vi "test4.3-AsyncMessageWithoutReply_Queue.vi"(8 "error in (no error)":errorcluster, 11 "TestCase in":refnum<class "testcase-CSMGlobalLog.lvclass">) -> (0 "error out":errorcluster, 3 "TestCase out":refnum<class "testcase-CSMGlobalLog.lvclass">)   [LabVIEW 2017, in "testcase-CSMGlobalLog.lvclass"]
uses:
  testcase-CSMGlobalLog.lvclass
  testcase-CSMGlobalLog.lvclass/testcase-CSMGlobalLog.ctl
  c9cb4a92-c6b2-48ff-9945-b938079fd949.vi
  <vilib>/addons/_JKI Toolkits/VI Tester/TestCase.llb/TestCase.lvclass
  src/user.lib/_NEVSTOP/Communicable State Machine(CSM)/Communicable State Machine.lvlib
  src/user.lib/_NEVSTOP/Communicable State Machine(CSM)/Utility/Periodic String Filter Setting.ctl
  C:/Program Files (x86)/National Instruments/LabVIEW 2017/vi.lib/addons/_JKI Toolkits/VI Tester/TestCase.llb/TestCase.lvclass
panel:
  out "String cache total":string
  out "LoopCount":i32
  out "String Cache each loop":string
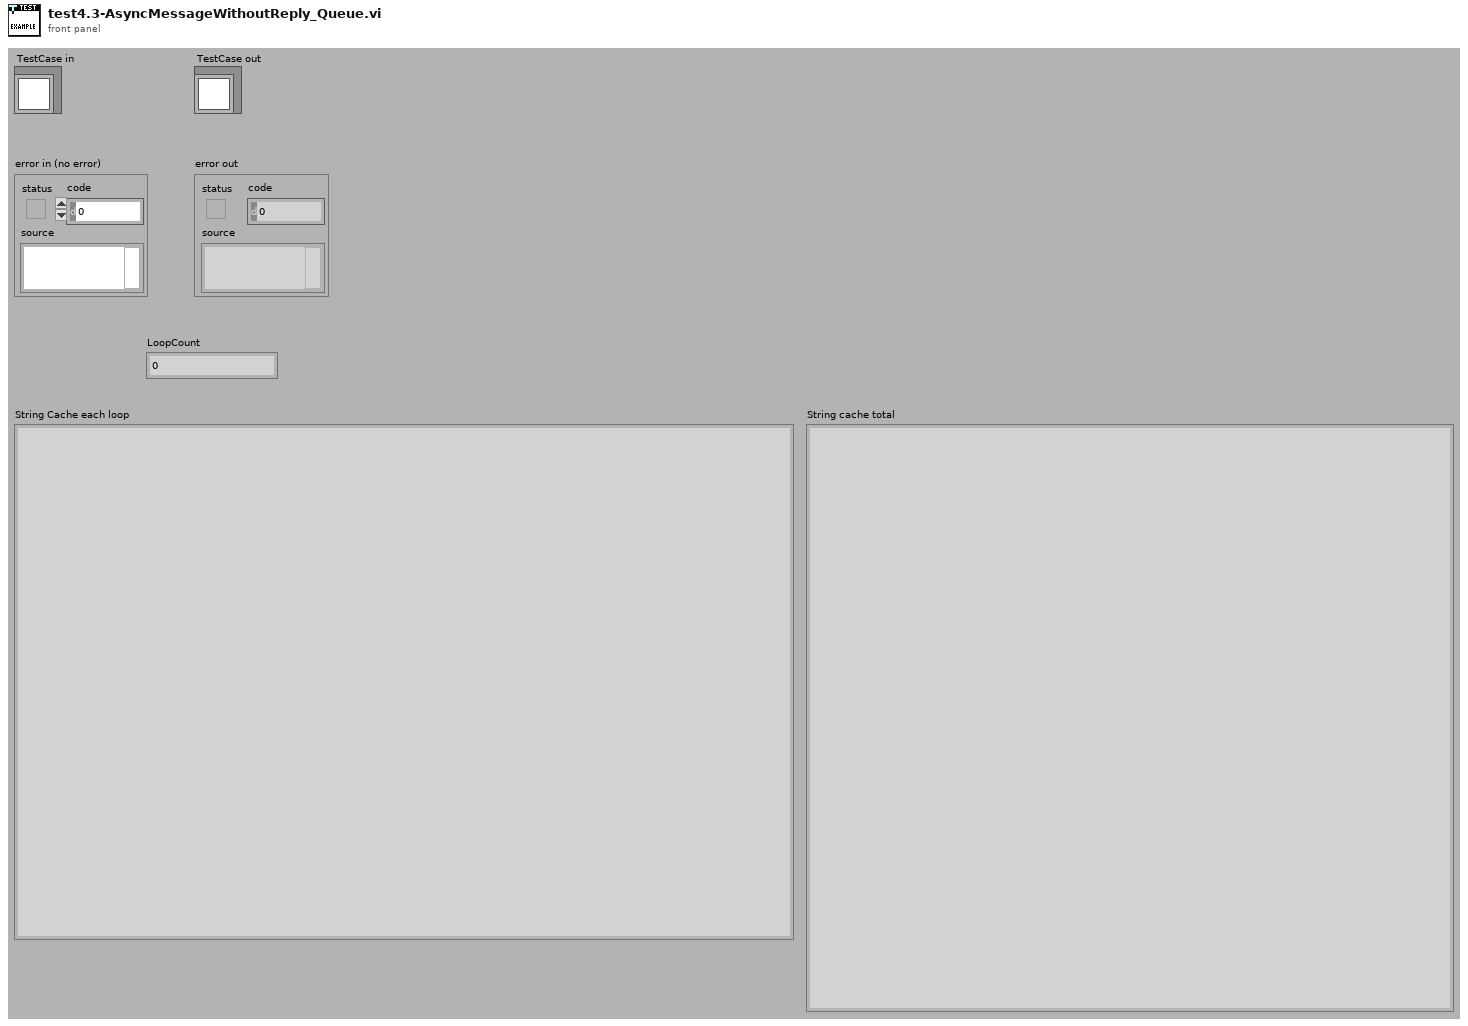
[diagram p1: front panel]
types:
  T1 = typedef "Communicable State Machine.lvlib/Periodic String Filter Setting.ctl" = cluster{"threashold(#/s)":dbl, "Check Peroid(s)":dbl}
  T2 = typedef "Communicable State Machine.lvlib/_CSM_GlobalLog_MSG.ctl" = cluster{"Name (\"\" to Use UUID)":string, "Current State":string, "Arguments":string, "Source Message":T3, "Source Module":string, "Complete(T)/Start(F)":bool, "LogType":T4, "Time Stamp":timestamp}
  T3 = typedef "Communicable State Machine.lvlib/_CSM_Response Source Message.ctl" = cluster{"‘State":string, "’Arguments":string, "’Error":errorcluster}
  T4 = typedef "Communicable State Machine.lvlib/_CSM_GlobalLog_MSG_TYPE.ctl" = enum16{"User Log", "State Change", "Status", "Interrupt", "Register", "Unregister", "Error Log", "Module Created", "Module Destroyed", "Async Message", "No-Rep Async Message", "Sync Message"}
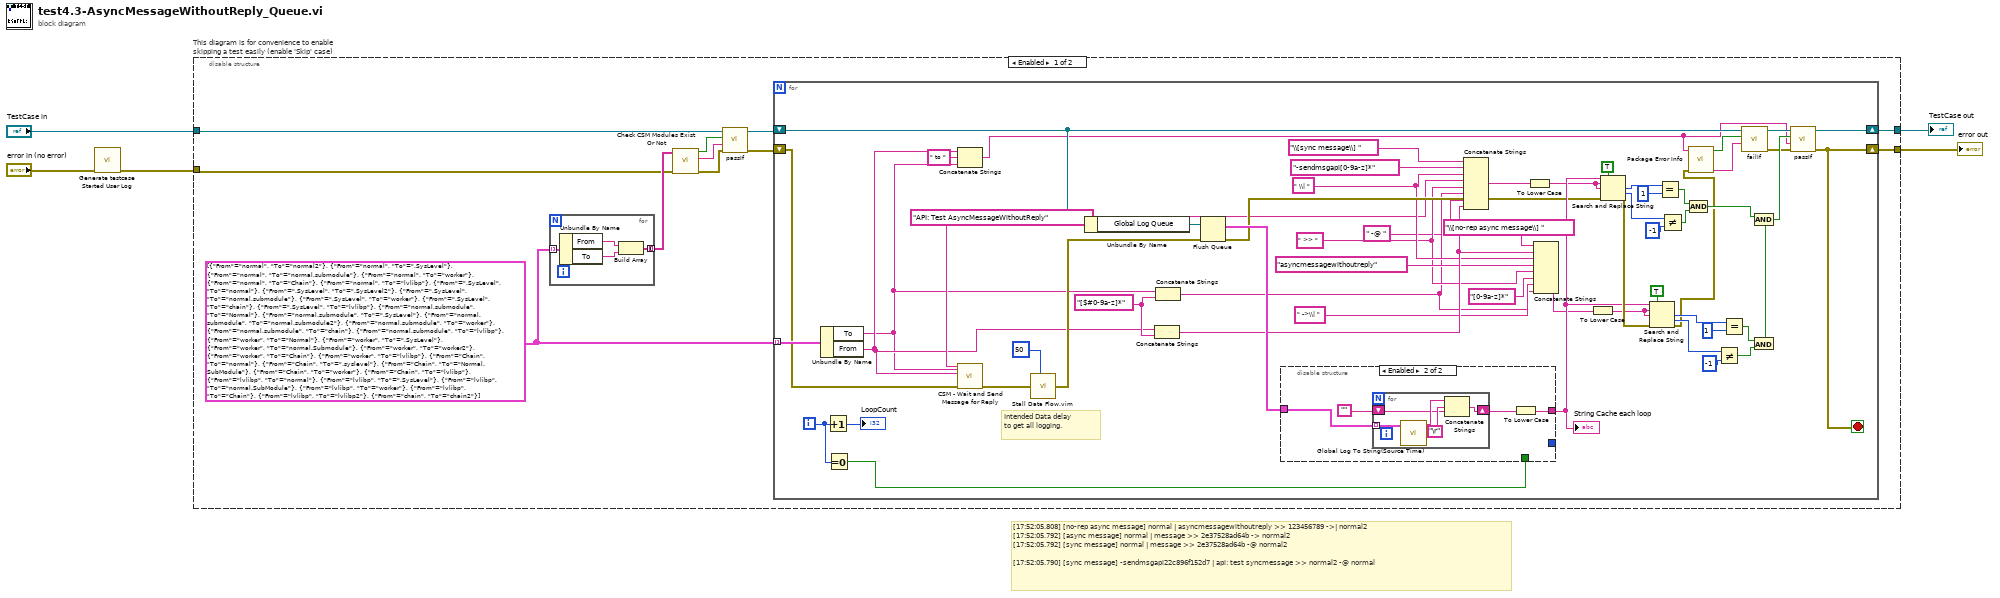
[diagram p0: block diagram]
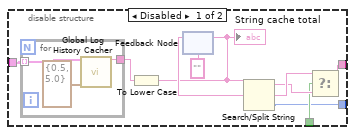
[diagram p2: hidden frame]
diagram:
  # "[17:52:05.808] [no-rep async message] normal | asyncmessagewithoutreply >> 123456789 ->| normal2\n[17:52:05.792] [async message] normal | message >> 2e37528ad64b -> normal2\n[17:52:05.792] [sync message] normal | message >> 2e37528ad64b -@ normal2\n\n[17:52:05.790] [sync message] -sendmsgapi22c896f152d7 | api: test syncmessage >> normal2 -@ normal"
  n1 = call "Generate testcase Started User Log.vi"("Error In"="error in (no error)") -> ("error out"=w1:errorcluster)  [unwired: 10 in]
  n2 = disable-structure "This diagram is for convenience to enable skipping a test easily (enable 'Skip' case)" shown="Enabled" {
    disable-tunnel: "TestCase in" -> [w9 w105]
    disable-tunnel: [w15 w103] -> w2
    disable-tunnel: [w16 w104] -> w4
    disable-tunnel: w1 -> [w6 w102]
    frame Enabled {
      w10 = cluster{"From":string, "To":string}[] [{"From"="normal", "To"="normal2"}, {"From"="normal", "To"=".SysLevel"}, {"From"="normal", "To"="normal.submodule"}, {"From"="normal", "To"="worker"}, {"From"="normal", "To"="Chain"}, {"From"="normal", "To"="lvlibp"}, {"From"=".SysLevel", "To"="normal"}, {"From"=".SysLevel", "To"=".SysLevel2"}, {"From"=".SysLevel", "To"="normal.submodule"}, {"From"=".SysLevel", "To"="worker"}, {"From"=".SysLevel", "To"="chain"}, {"From"=".SysLevel", "To"="lvlibp"}, {"From"="normal.submodule", "To"="Normal"}, {"From"="normal.submodule", "To"=".SysLevel"}, {"From"="normal.submodule", "To"="normal.submodule2"}, {"From"="normal.submodule", "To"="worker"}, {"From"="normal.submodule", "To"="chain"}, {"From"="normal.submodule", "To"="lvlibp"}, {"From"="worker", "To"="Normal"}, {"From"="worker", "To"=".SysLevel"}, {"From"="worker", "To"="normal.Submodule"}, {"From"="worker", "To"="worker2"}, {"From"="worker", "To"="Chain"}, {"From"="worker", "To"="lvlibp"}, {"From"="Chain", "To"="normal"}, {"From"="Chain", "To"=".syslevel"}, {"From"="Chain", "To"="Normal.SubModule"}, {"From"="Chain", "To"="worker"}, {"From"="Chain", "To"="lvlibp"}, {"From"="lvlibp", "To"="normal"}, {"From"="lvlibp", "To"=".SysLevel"}, {"From"="lvlibp", "To"="normal.SubModule"}, {"From"="lvlibp", "To"="worker"}, {"From"="lvlibp", "To"="Chain"}, {"From"="lvlibp", "To"="lvlibp2"}, {"From"="chain", "To"="chain2"}]
      n3 = for {
        tunnel: w10 -> [w20] mode=indexing
        tunnel: [w17] -> w13 mode=concatenating
        n4 = Unbundle By Name(w20) -> ("From"=w19:string, "To"=w18:string)
        n5 = Build Array(w19, w18) -> (w17:string[])
      }
      n6 = call "Check CSM Modules Exist Or Not.vi"("error in"=w6, "CSM names in"=w13) -> ("error out"=w11:errorcluster, "Debug string"=w12:string, "All Modules Exist?"=w14:bool)  [unwired: 7 in]
      n7 = call-dynamic "passIf.vi"("error in (no error)"=w11, "message (\"\")"=w12, "pass"=w14, "TestCase in"=w9) -> ("error out"=w7:errorcluster, "TestCase out"=w8:refnum<class "testcase-CSMGlobalLog.lvclass">)  [unwired: 6 in]
      n8 = for {
        tunnel: w10 -> [w59] mode=indexing
        shift-right: [w58] -> w16
        shift-left: w7 -> [w31]
        shift-right: [w79] -> w15
        shift-left: w8 -> [w28]
        i -> [w57]
        stop <- w58 stop-if-true
        w33 = "[$#0-9a-z]*" ("string")
        w43 = " >> "
        w45 = " \\| "
        w35 = "API: Test AsyncMessageWithoutReply" ("State")
        # "Intended Data delay\nto get all logging."
        n9 = Unbundle By Name(w59) -> ("To"=w23:string, "From"=w24:string)
        n10 = Increment(x=w57) -> (x+1=→"LoopCount":i32)
        n11 = Equal To 0?(x=w57) -> (x = 0?=w50:bool)
        n12 = Concatenate Strings(w24, " to " ("string"), w23) -> (w21:string)
        n13 = call "CSM - Wait and Send Message for Reply.vi"("State"=w35, "Arguments (\"\")"=w23, "Target Module"=w24, "Error In (No Error)"=w31) -> ("error out"=w56:errorcluster)  [unwired: 8 in, 3 out]
        n14 = call "Stall Data Flow.vim"("value in"=w56, "milliseconds to wait"=u32 50 ("millisecond timer value")) -> ("value out"=w55:errorcluster)  [unwired: 1 out]
        n15 = Unbundle By Name(w28) -> ("Global Log Queue"=w78:refnum<queue>)
        n16 = Concatenate Strings(w24, w33) -> (w46:string)
        n17 = Concatenate Strings(w23, w33) -> (w40:string)
        n18 = Flush Queue(queue=w78, error in (no error)=w55) -> (remaining elements=w52:T2[], error out=w49:errorcluster)  [unwired: 1 out]
        n19 = disable-structure shown="Enabled" {
          disable-tunnel: [w83 w93] -> w51
          disable-tunnel: w50 -> [w82 _]
          disable-tunnel: w52 -> [w81 w95]
          disable-tunnel: [w80 _] -> _
          frame Disabled {
            n20 = for {
              tunnel: w81 -> [w92] mode=indexing
              tunnel: [w91] -> w89
              n21 = call "Global Log History Cacher.vi"("Global Log Data"=w92, "Settings"=T1 {"threashold(#/s)"=0.5, "Check Peroid(s)"=5.0}) -> ("String Cache"=w91:string)  [unwired: 13 in]
            }
            n22 = To Lower Case(string=w89) -> (all lower case string=w84:string)
            "String cache total" <- w84
            n23 = feedback #1("") -> (w88:string)
            n24 = feedback-in #1(w84) -> ()
            n25 = Search/Split String(string=w84, search string/char (-)=w88) -> (substring before match=w85:string, match + rest of string=w86:string, offset of match=w80:i32)  [unwired: 1 in]
            n26 = Select(t=w86, s=w82, f=w85) -> (s? t:f=w83:string)
          }
          frame Enabled {
            n27 = for {
              tunnel: w95 -> [w101] mode=indexing
              shift-right: [w97] -> w94
              shift-left: "" -> [w98]
              n28 = call "Global Log To String(Source Time).vi"("Log"=w101) -> ("Log String"=w100:string)  [unwired: 9 in]
              n29 = Concatenate Strings(w100, "\r", w98) -> (w97:string)
            }
            n30 = To Lower Case(string=w94) -> (all lower case string=w93:string)
          }
        }
        "String Cache each loop" <- w51
        n31 = Concatenate Strings("\\[sync message\\] ", "-sendmsgapi[0-9a-z]*", w45, w35, w43, w40, " -@ " ("string"), w46) -> (w39:string)
        n32 = To Lower Case(string=w39) -> (all lower case string=w38:string)
        n33 = Concatenate Strings("\\[no-rep async message\\] " ("string"), w46, w45, "asyncmessagewithoutreply", w43, "[0-9a-z]*", " ->\\| ", w40) -> (w37:string)
        n34 = To Lower Case(string=w37) -> (all lower case string=w36:string)
        n35 = Search and Replace String(replace all?=TRUE ("replace all? (F)"), input string=w51, search string=w38, replace string=w38, error in=w49) -> (number of replacements=w75:i32, offset past replacement=w74:i32, error out=w64:errorcluster)  [unwired: 3 in, 1 out]
        n36 = Search and Replace String(replace all?=TRUE ("replace all? (F)"), input string=w51, search string=w36, replace string=w36, error in=w64) -> (number of replacements=w66:i32, offset past replacement=w67:i32, error out=w25:errorcluster)  [unwired: 3 in, 1 out]
        n37 = Equal?(x=w75, y=1) -> (x = y?=w72:bool)
        n38 = Not Equal?(x=w74, y=-1) -> (x != y?=w71:bool)
        n39 = And(x=w72, y=w71) -> (x .and. y?=w60:bool)
        n40 = call "Package Error Info.vi"("error in"=w25, "String in"=w21) -> ("packed error info out"=w29:string, "error status"=w30:bool)  [unwired: 8 in]
        n41 = Not Equal?(x=w67, y=-1) -> (x != y?=w70:bool)
        n42 = Equal?(x=w66, y=1) -> (x = y?=w69:bool)
        n43 = call-dynamic "failIf.vi"("message (\"\")"=w29, "fail"=w30, "TestCase in"=w28) -> ("error out"=w26:errorcluster, "TestCase out"=w27:refnum<class "testcase-CSMGlobalLog.lvclass">)  [unwired: 7 in]
        n44 = And(x=w69, y=w70) -> (x .and. y?=w63:bool)
        n45 = And(x=w60, y=w63) -> (x .and. y?=w53:bool)
        n46 = call-dynamic "passIf.vi"("error in (no error)"=w26, "message (\"\")"=w21, "pass"=w53, "TestCase in"=w27) -> ("error out"=w58:errorcluster, "TestCase out"=w79:refnum<class "testcase-CSMGlobalLog.lvclass">)  [unwired: 6 in]
      }
    }
    frame Disabled {
      # "skip test result while test is under development"
      n47 = call <vilib>:"skip.vi"("error in (no error)"=w102, "TestCase in"=w105) -> ("error out"=w104:errorcluster, "TestCase out"=w103:refnum<class "testcase-CSMGlobalLog.lvclass">)  [unwired: 8 in]
    }
  }
  "error out" <- w4
  "TestCase out" <- w2
